vi "fg_file.vi"(8 "error in (no error)":errorcluster, 11 "file":T1) -> (0 "error out":errorcluster, 3 "filename":path)   [LabVIEW 2015, in "lv-bin-template.lvlib"]
uses:
  lv-bin-template.lvlib
  _control/file.ctl
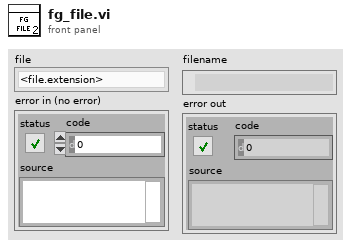
[diagram p1: front panel]
types:
  T1 = typedef "lv-bin-template.lvlib/file.ctl" = enum16{"<file.extension>"}
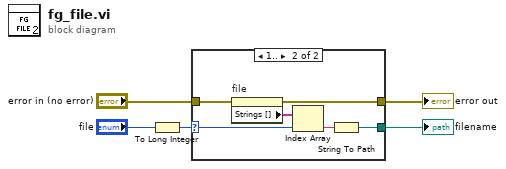
[diagram p0: block diagram]
diagram:
  n1 = To Long Integer(number="file") -> (32bit integer=w4:i32)
  n2 = case shown="1.." w4 {
    selector: w4 -> [_ w7]
    tunnel: "error in (no error)" -> [w6 w12]
    tunnel: [w6 w11] -> w1
    tunnel: [_ w8] -> w2
    frame Default {
    }
    frame 1.. {
      n3 = property on="file" class="Enum (strict)"(error in=w12) -> (error out=w11:errorcluster, "Strings []"=w10:string[])  [unwired: 1 in, 1 out]
      n4 = Index Array(array=w10, index=w7) -> (element=w9:string)
      n5 = String To Path(string=w9) -> (path=w8:path)
    }
  }
  "filename" <- w2
  "error out" <- w1
